vi "AverageXYZNew (SubVI).vi"(8 "array":dbl[][][](array[numeric])=[[[-616.6853013924161, 133.98498133920288, 23.19072534]], [[-602.0918631529712, 134.0873275784507, 23.19072534]], [[-616.6844686564219, 133.98510562595666, 23.19072534]], [[-602.0873483929206, 134.10375101417594, 23.19072534]], [[-616.6848465163853, 133.9845728817171, 23.19072534]], [[-602.0884296079262, 134.087169544694, 23.19072534]], [[-334.3899800940794, 135.67998739590436, 23.19072534]], [[-323.9779865268114, 134.48344180918818, 23.19072534]], [[-334.3927140881534, 135.68204709551367, 23.19072534]], [[-323.98295164227596, 134.48329915078338, 23.19072534]], [[-334.3923216504359, 135.6810484407434, 23.19072534]], [[-323.97787795641597, 134.480380149028, 23.19072534]], [[-40.3112304344497, 135.51048660072627, 23.19072534]], [[-29.903300498442807, 134.22953193062764, 23.19082534]], [[-40.31259391421408, 135.5137627222535, 23.19072534]], [[-29.90268539871824, 134.2294673759651, 23.19072534]], [[-40.309615844169045, 135.51088795666246, 23.19072534]], [[-29.90442472417554, 134.2282083267235, 23.19072534]], [[253.79560124818477, 135.34840869395944, 23.19082534]], [[264.2326481830148, 134.22077460141287, 23.19082534]], [[253.79296388701863, 135.34828494250544, 23.19072534]], [[264.2354027367716, 134.217503625029, 23.19072534]], [[253.79395739751806, 135.34811629532663, 23.19072534]], [[264.23504153416127, 134.2164607476983, 23.19072534]]], 10 "Number of images each":i32=3, 11 "Number of pins":i32=4) -> (2 "Uncertainty":dbl[][](array[numeric])=[[7.994371529286357, 5.702924101377151, 5.700519308587177, 5.718327693690156], [0.05938566398452695, 0.6565310349097196, 0.7025336898765229, 0.618941088980328], [0.0, 0.0, 4.082482904629116e-05, 5.1639777949311874e-05]], 3 "Averages":dbl[][](array[numeric])=[[-609.3870429531735, -329.18563865969537, -35.10730846902823, 259.01426916444484], [134.0388179973662, 135.08170067352683, 134.8703908188264, 134.78325815098862], [23.19072534, 23.19072534, 23.190742006666667, 23.190758673333335]])   [LabVIEW 2016]
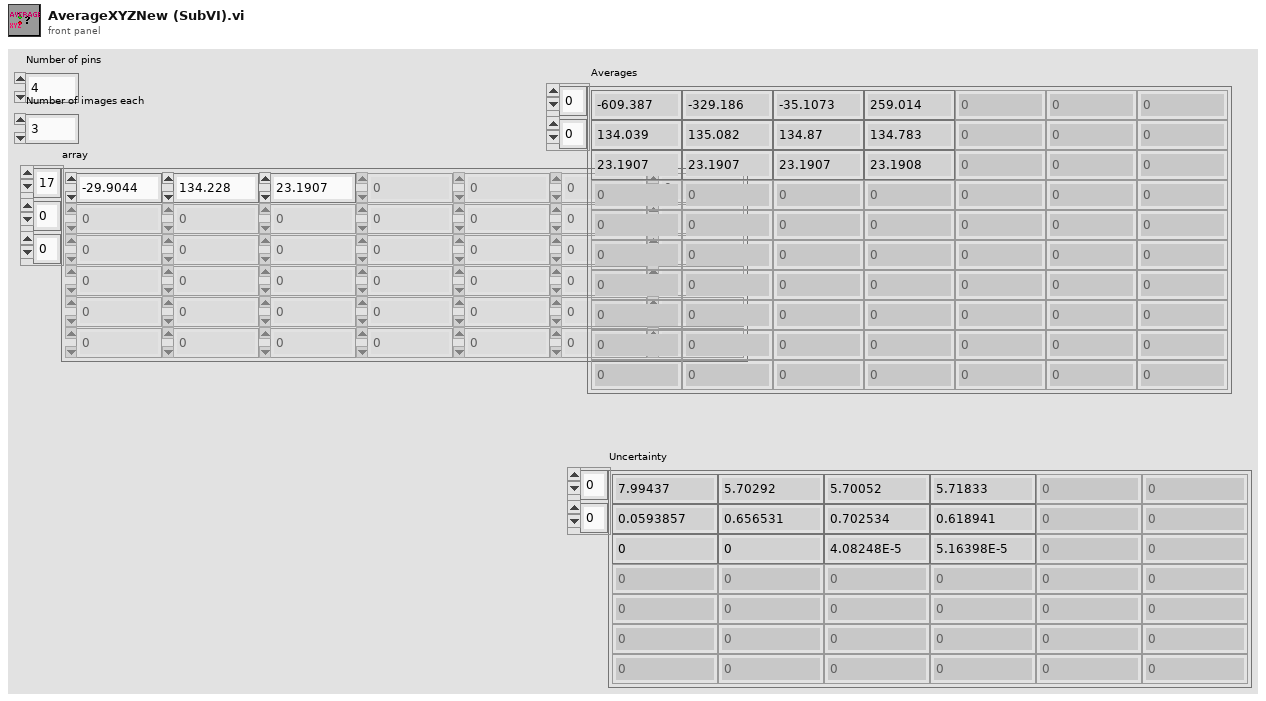
[diagram p1: front panel]
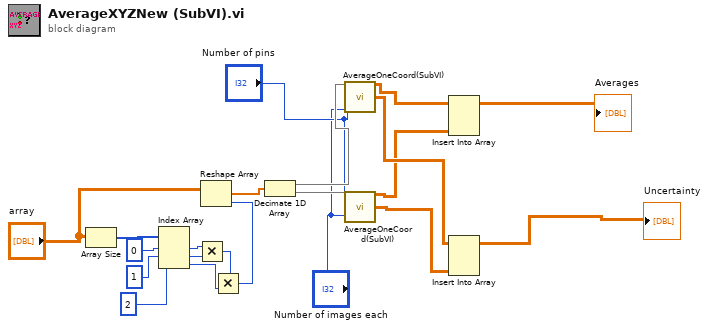
[diagram p0: block diagram]
diagram:
  n1 = Array Size(array="array") -> (size(s)=w21:i32[])
  n2 = Index Array(array=w21, index #1=0 ("index"), index #2=1 ("index"), index #3=2 ("index")) -> (element #1=w18:i32, element #2=w17:i32, element #3=w3:i32)
  n3 = Multiply(x=w18, y=w17) -> (x*y=w2:i32)
  n4 = Multiply(x=w2, y=w3) -> (x*y=w1:i32)
  n5 = Reshape Array("array", w1) -> (w15:dbl[])
  n6 = Decimate 1D Array(w15) -> (w14:dbl[], w11:dbl[])
  n7 = call "AverageOneCoord(SubVI).vi"("Array"=w14, "Number of pins"="Number of pins", "Number of images each"="Number of images each") -> ("Averages"=w13:dbl[][], "SD"=w12:dbl[][])  [unwired: 11 in]
  n8 = call "AverageOneCoord(SubVI).vi"("Array"=w11, "Number of pins"="Number of pins", "Number of images each"="Number of images each") -> ("Averages"=w10:dbl[][], "SD"=w9:dbl[][])  [unwired: 11 in]
  n9 = Insert Into Array(array=w13, new element=w10) -> (→"Averages":dbl[][])  [unwired: 2 in]
  n10 = Insert Into Array(array=w12, new element=w9) -> (→"Uncertainty":dbl[][])  [unwired: 2 in]
